vi "menu-ReplaceSeperatorWith---.vi"(11 "Array in":T1[](array[typedef])) -> (3 "Array out":T1[](array[typedef]))   [LabVIEW 2019]
uses:
  <resource>/Framework/Providers/API/mxLvMenuItem.ctl
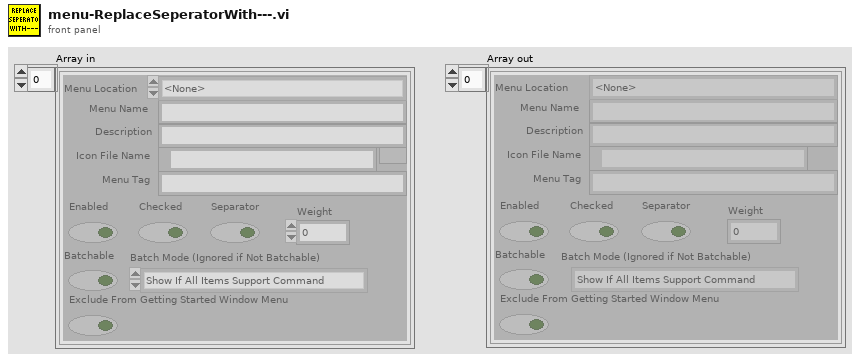
[diagram p1: front panel]
types:
  T1 = typedef "mxLvMenuItem.ctl" = cluster{"Menu Name":string, "Description":string, "Icon File Name":path, "Menu Tag":string, "Enabled":bool, "Checked":bool, "Separator":bool, "Batchable":bool, "Weight":i32, "Batch Mode (Ignored if Not Batchable)":enum32{"Show If All Items Support Command", "Show If Any Items Support Command"}, "Menu Location":enum32{"<None>", "Project", "Project / Build Specifications", "Tools", "Tools / Source Control", "Tools / Real-Time Module", "Help"}, "Exclude From Getting Started Window Menu":bool}
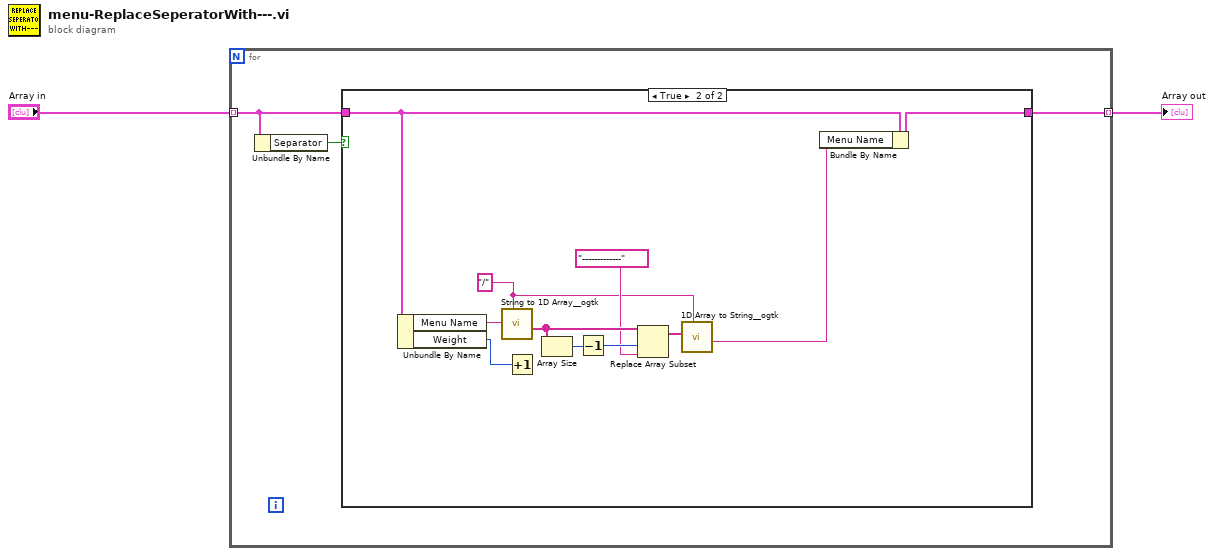
[diagram p0: block diagram]
diagram:
  n1 = for {
    tunnel: "Array in" -> [w4] mode=indexing
    tunnel: [w5] -> w1 mode=indexing
    n2 = Unbundle By Name(w4) -> ("Separator"=w3:bool)
    n3 = case shown="True" w3 {
      tunnel: [w6 w17] -> w5
      tunnel: w4 -> [w6 w8]
      frame False {
      }
      frame True {
        w9 = "/" ("delimiter (Tab)")
        n4 = Unbundle By Name(w8) -> ("Menu Name"=w15:string, "Weight"=w16:i32)
        n5 = call <userlib>:"String to 1D Array__ogtk.vi"("delimiter (Tab)"=w9, "string"=w15) -> ("Array of Strings"=w13:string[])  [unwired: 9 in]
        n6 = Increment(x=w16) -> ()  [unwired: 1 out]
        n7 = Array Size(array=w13) -> (size(s)=w14:i32)
        n8 = Decrement(x=w14) -> (x-1=w12:i32)
        n9 = Replace Array Subset(array=w13, new element="-------------" ("delimiter (Tab)"), index=w12) -> (w10:string[])
        n10 = call <userlib>:"1D Array to String__ogtk.vi"("delimiter (Tab)"=w9, "Array of Strings"=w10) -> ("delimited string"=w7:string)  [unwired: 9 in]
        n11 = Bundle By Name(cluster=w8, "Menu Name"=w7) -> (w17:T1)
      }
    }
  }
  "Array out" <- w1
